vi "Process TWM result.vi"(6 "Quantity to read":string="rms", 8 "error from TWM get result":errorcluster, 9 "Calculate RMS from samples":bool, 10 "TWM result":T1[][](array[typedef])) -> (0 "error out":errorcluster, 2 "TWM result as number":dbl[][](array[numeric]), 3 "TWM result as string":string[][](array[string]))   [LabVIEW 2020]
doc: "Obtain TWM result. If no calculation set, result is N/A. If calculation error, result is Err."
uses:
  external libraries/TWM-1.8.7.0-client/TWM Client Quantity Record.ctl
  external libraries/TWM-1.8.7.0-client/TWM Client.lvlib
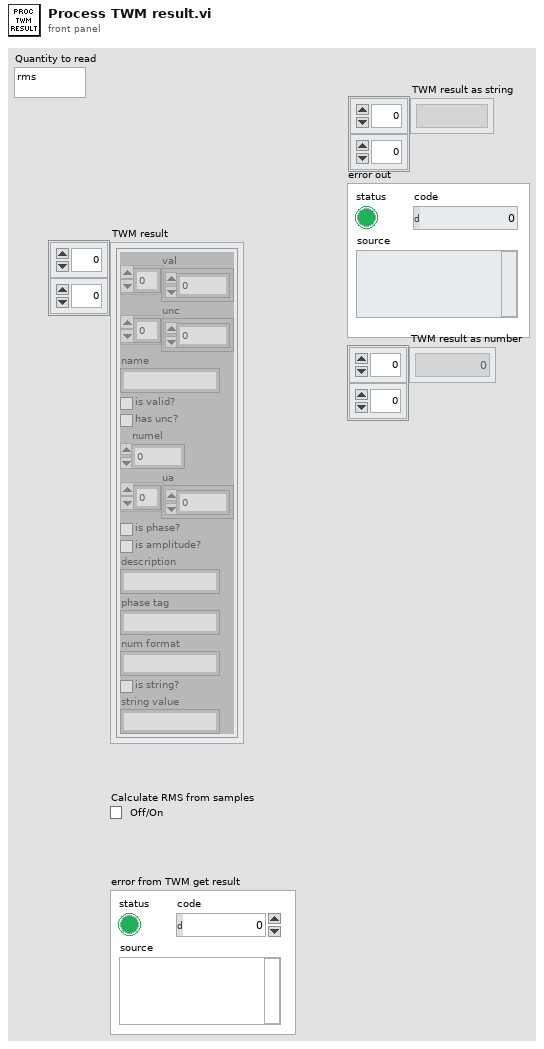
[diagram p1: front panel]
types:
  T1 = typedef "TWM Client.lvlib/TWM Client Quantity Record.ctl" = cluster{"val":dbl[], "unc":dbl[], "name":string, "is valid?":bool, "has unc?":bool, "numel":i32, "ua":dbl[], "is phase?":bool, "is amplitude?":bool, "description":string, "phase tag":string, "num format":string, "is string?":bool, "string value":string}
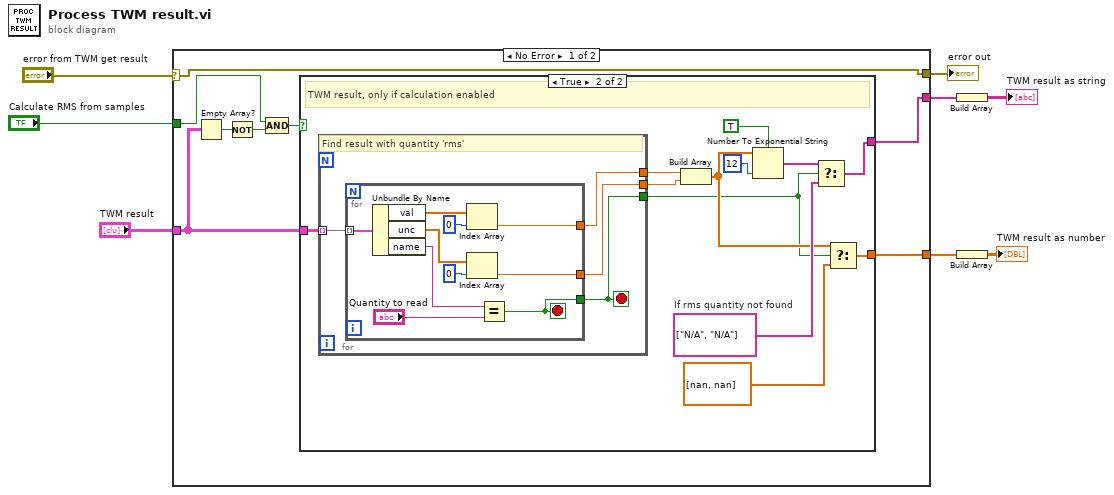
[diagram p0: block diagram]
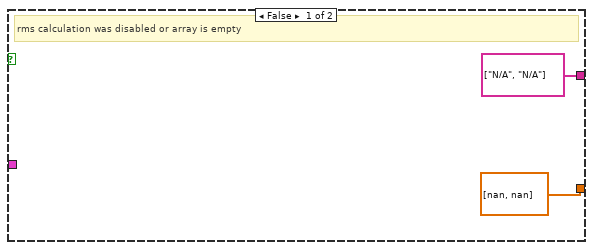
[diagram p2: hidden frame]
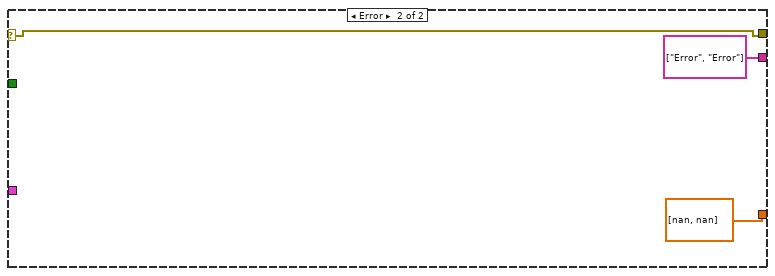
[diagram p3: hidden frame]
diagram:
  n1 = case shown="No Error" "error from TWM get result" {
    selector: "error from TWM get result" -> [w10 w46]
    tunnel: "Calculate RMS from samples" -> [w13 _]
    tunnel: "TWM result" -> [w15 _]
    tunnel: [w16 string[] ["Error", "Error"] ("f")] -> w6
    tunnel: [w10 w46] -> w4
    tunnel: [w9 dbl[] [nan, nan]] -> w2
    frame No Error {
      n2 = Empty Array?(array=w15) -> (empty?=w12:bool)
      n3 = Not(x=w12) -> (.not. x?=w11:bool)
      n4 = Compound Arithmetic op=AND(w13, w11) -> (w14:bool)
      n5 = case shown="True" w14 {
        tunnel: w15 -> [_ w30]
        tunnel: [string[] ["N/A", "N/A"] ("f") w23] -> w16
        tunnel: [dbl[] [nan, nan] w19] -> w9
        frame False {
          # "rms calculation was disabled or array is empty"
        }
        frame True {
          w24 = string[] ["N/A", "N/A"]  # If rms quantity not found
          # "TWM result, only if calculation enabled"
          n6 = for {
            tunnel: w30 -> [w34] mode=indexing
            tunnel: [w33] -> w28
            tunnel: [w32] -> w29
            tunnel: [w31] -> w20
            stop <- w31 stop-if-true
            # "Find result with quantity 'rms'"
            n7 = for {
              tunnel: w34 -> [w44] mode=indexing
              tunnel: [w42] -> w31
              tunnel: [w40] -> w33
              tunnel: [w36] -> w32
              stop <- w42 stop-if-true
              n8 = Unbundle By Name(w44) -> ("val"=w41:dbl[], "unc"=w37:dbl[], "name"=w43:string)
              n9 = Index Array(array=w41, index=0) -> (element=w40:dbl)
              n10 = Index Array(array=w37, index=0) -> (element=w36:dbl)
              n11 = Equal?(x=w43, y="Quantity to read") -> (x = y?=w42:bool)
            }
          }
          n12 = Build Array(w28, w29) -> (w21:dbl[])
          n13 = Number To Exponential String(number=w21, precision (6)=i16 12, 1:TRUE ("use system decimal point (T)")) -> (E-format string=w25:string[])  [unwired: 1 in]
          n14 = Select(t=w25, s=w20, f=w24) -> (s? t:f=w23:string[])
          n15 = Select(t=w21, s=w20, f=dbl[] [nan, nan]) -> (s? t:f=w19:dbl[])
        }
      }
    }
    frame Error {
    }
  }
  "error out" <- w4
  n16 = Build Array(w6) -> (→"TWM result as string":string[][])
  n17 = Build Array(w2) -> (→"TWM result as number":dbl[][])
